vi "NML GPIB Data Log.vi"(0 "Point #":i32) -> (1 "GPIB Data":dbl[](array[numeric]) format="%.4e", 2 "Stop":bool)   [LabVIEW 2019]
doc: "VI which calls the appropriate GPIB routines for a variety of instruments.\nScott Hannahs, NHMFL-FSU, Nov. 1993"
uses:
  Sub Controls/Instrument.ctl
  Sub Controls/NML GPIB List.ctl
panel:
  in  "GPIB settings":T3={"#1"={"Instrument"=enum."None", "Instrument Address"="", "Parameters"=[]}, "#2"={"Instrument"=enum."None", "Instrument Address"="", "Parameters"=[]}, "#3"={"Instrument"=enum."None", "Instrument Address"="", "Parameters"=[]}, "#4"={"Instrument"=enum."None", "Instrument Address"="", "Parameters"=[]}, "#5"={"Instrument"=enum."None", "Instrument Address"="", "Parameters"=[]}, "#6"={"Instrument"=enum."None", "Instrument Address"="", "Parameters"=[]}, "#7"={"Instrument"=enum."None", "Instrument Address"="", "Parameters"=[]}, "#8"={"Instrument"=enum."None", "Instrument Address"="", "Parameters"=[]}, "#9"={"Instrument"=enum."None", "Instrument Address"="", "Parameters"=[]}, "#10"={"Instrument"=enum."None", "Instrument Address"="", "Parameters"=[]}, "#11"={"Instrument"=enum."None", "Instrument Address"="", "Parameters"=[]}, "#12"={"Instrument"=enum."None", "Instrument Address"="", "Parameters"=[]}, "#13"={"Instrument"=enum."None", "Instrument Address"="", "Parameters"=[]}, "#14"={"Instrument"=enum."None", "Instrument Address"="", "Parameters"=[]}, "#15"={"Instrument"=enum."None", "Instrument Address"="", "Parameters"=[]}, "#16"={"Instrument"=enum."None", "Instrument Address"="", "Parameters"=[]}, "#17"={"Instrument"=enum."None", "Instrument Address"="", "Parameters"=[]}, "#18"={"Instrument"=enum."None", "Instrument Address"="", "Parameters"=[]}, "#19"={"Instrument"=enum."None", "Instrument Address"="", "Parameters"=[]}, "#20"={"Instrument"=enum."Time Stamp", "Instrument Address"="", "Parameters"=[]}} {"#16"."Parameters" format="%.3e"; "#20"."Parameters" format="%.3e"; "#18"."Parameters" format="%.3e"; "#17"."Parameters" format="%.3e"; "#19"."Parameters" format="%.3e"; "#11"."Parameters" format="%.3e"; "#15"."Parameters" format="%.3e"; "#13"."Parameters" format="%.3e"; "#12"."Parameters" format="%.3e"; "#14"."Parameters" format="%.3e"; "#6"."Parameters" format="%.3e"; "#10"."Parameters" format="%.3e"; "#8"."Parameters" format="%.3e"; "#7"."Parameters" format="%.3e"; "#9"."Parameters" format="%.3e"; "#1"."Parameters" format="%.3e"; "#5"."Parameters" format="%.3e"; "#3"."Parameters" format="%.3e"; "#2"."Parameters" format="%.3e"; "#4"."Parameters" format="%.3e"}
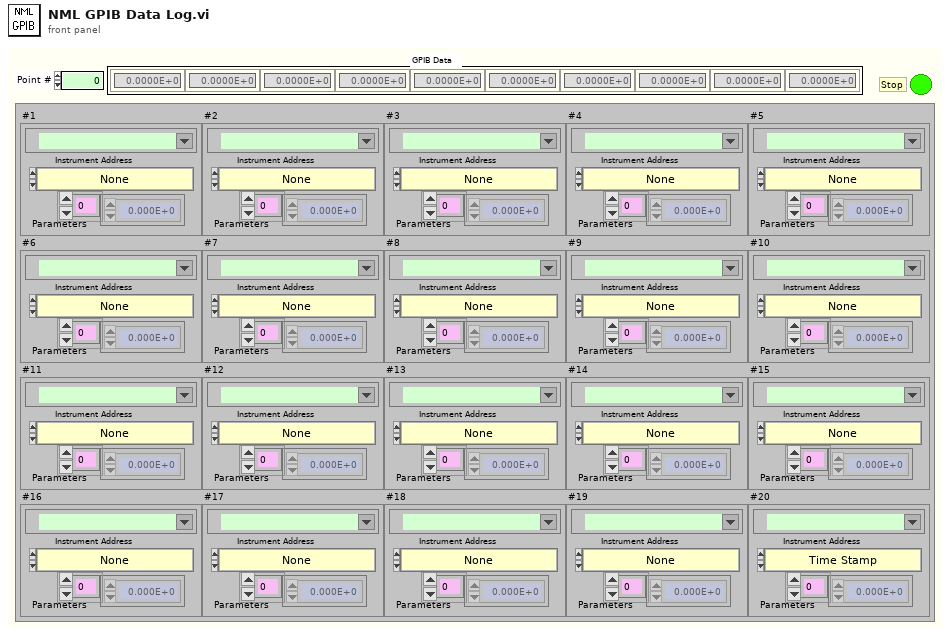
[diagram p1: front panel]
types:
  T1 = typedef "Instrument.ctl" = cluster{"Instrument":T2, "Instrument Address":refnum<visa-resource-name>, "Parameters":dbl[]}
  T2 = typedef "NML GPIB List.ctl" = enum16{"None", "Field", "Field - SCM1", "DMM", "DMM - HP 34401", "Keithley 2XXX", "Running DMM Ave", "Running HP34401", "Running K2XXX Ave", "SRS 830 - CH 1", "SRS 830 - CH1 & 2", "SRS PTC10", "Signal Rec 7265 - X", "Signal Rec 7265 - X&Y", "DRC 93C - Sample", "DRC 93C - Control", "DRC 93C - Sam&Con", "CryoCon Sensor A", "CryoCon Sensor B", "Cond 20C Sensor 1", "Cond 20C Sensor 2", "LS 336 Read", "LS 340 Read", "LS 370 Read", "LS 370 Select", "AVS 46 Bridge", "BLM Rotator Read Position", "Linear Research 700", "LR 700 Select", "Keithley 3330 - LCZ", "A-H Capacitance", "Digital Integrator", "SRS 400 Phot Ctr", "LakeShore VSM", "AMI He Level Meter", "Time Stamp", "Wait", "Invert Current", "K230 Linear V", "K230 VÅB^2", "Temp Ramp", "Power Ramp", "Freq Sweep", "LTC Stable T", "Scanner Step", "IMS Stepper Increment", "BLM Stepper Increment", "Omega CNi32"}
  T3 = cluster{"#1":T1, "#2":T1, "#3":T1, "#4":T1, "#5":T1, "#6":T1, "#7":T1, "#8":T1, "#9":T1, "#10":T1, "#11":T1, "#12":T1, "#13":T1, "#14":T1, "#15":T1, "#16":T1, "#17":T1, "#18":T1, "#19":T1, "#20":T1}
  T4 = cluster{"[0]":T1, "[1]":T1, "[2]":T1, "[3]":T1, "[4]":T1, "[5]":T1, "[6]":T1, "[7]":T1, "[8]":T1, "[9]":T1, "[10]":T1, "[11]":T1, "[12]":T1, "[13]":T1, "[14]":T1, "[15]":T1, "[16]":T1, "[17]":T1, "[18]":T1, "[19]":T1}
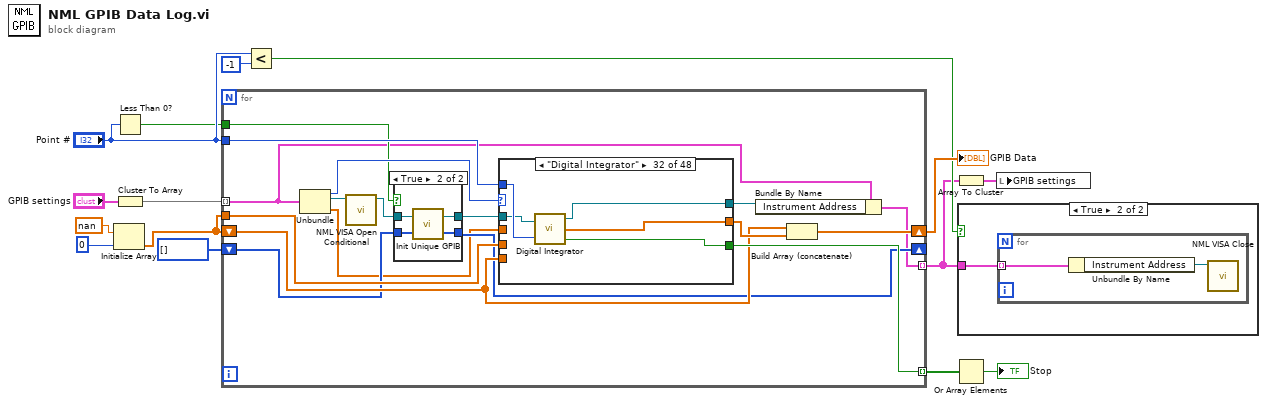
[diagram p0: block diagram]
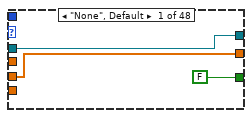
[diagram p4: hidden frame]
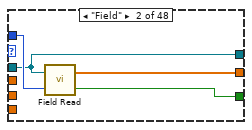
[diagram p5: hidden frame]
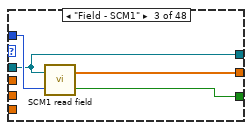
[diagram p6: hidden frame]
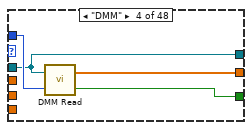
[diagram p7: hidden frame]
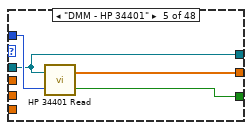
[diagram p8: hidden frame]
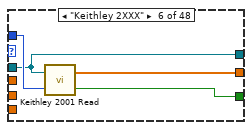
[diagram p9: hidden frame]
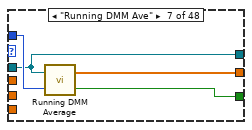
[diagram p10: hidden frame]
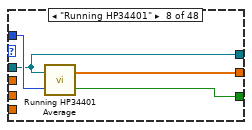
[diagram p11: hidden frame]
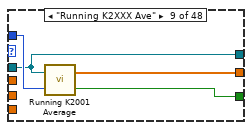
[diagram p12: hidden frame]
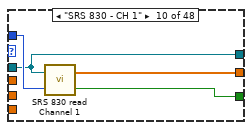
[diagram p13: hidden frame]
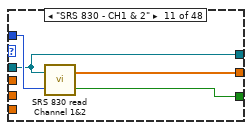
[diagram p14: hidden frame]
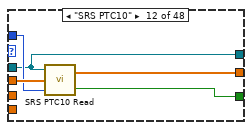
[diagram p15: hidden frame]
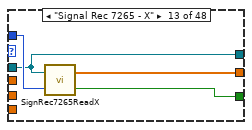
[diagram p16: hidden frame]
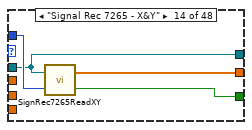
[diagram p17: hidden frame]
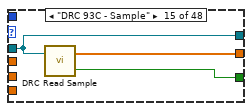
[diagram p18: hidden frame]
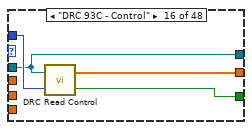
[diagram p19: hidden frame]
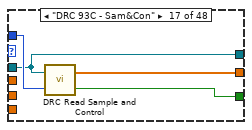
[diagram p20: hidden frame]
diagram:
  n1 = Initialize Array(nan, 0) -> (w5:dbl[])
  n2 = Less Than 0?(x="Point #") -> (x < 0?=w4:bool)
  n3 = Cluster To Array(cluster="GPIB settings") -> (array=w12:T1[])
  n4 = for {
    shift-right: [w32] -> w15
    shift-left: w5 -> [w27]
    tunnel: "Point #" -> [w23]
    tunnel: w12 -> [w21] mode=indexing
    tunnel: [w29] -> w11 mode=indexing
    tunnel: w5 -> [w28]
    tunnel: w4 -> [w22]
    shift-right: [w25] -> _
    shift-left: u16[] [] ("Inited dup") -> [w26]
    tunnel: [w20] -> w1 mode=indexing
    n5 = Unbundle(w21) -> ("Instrument"=w30:T2, "Instrument Address"=w16:refnum<visa-resource-name>, "Parameters"=w24:dbl[])
    n6 = call "NML VISA Open Conditional.vi"("VISA resource name"=w16) -> ("dup VISA Session"=w17:refnum<visa-resource-name>)  [unwired: 8 in, 2 out]
    n7 = case shown="True" w22 {
      tunnel: w26 -> [w33 w38]
      tunnel: [w33 w37] -> w25
      tunnel: w17 -> [w34 w36]
      tunnel: [w34 w35] -> w19
      frame False {
      }
      frame True {
        n8 = call "Init Unique GPIB.vi"("Inited"=w38, "VISA resource name"=w36) -> ("Inited dup"=w37:u16[], "dup VISA resource"=w35:refnum<visa-resource-name>)
      }
    }
    n9 = case shown="\"Digital Integrator\"" w30 {
      tunnel: [FALSE w44 w48 w52 w56 w60 w64 w68 w72 w77 w81 w83 w89 w93 w97 w101 w105 w108 w112 w116 w120 w124 w130 w135 w140 FALSE ("Stop") w149 w152 w156 w159 w163 w166 w172 w175 w179 w182 w187 w192 w197 w202 w207 w212 w217 w219 w225 w231 w233 w239] -> w29
      tunnel: w23 -> [_ w43 w47 w51 w55 w59 w63 w67 w71 w75 w79 w85 w88 w92 _ w99 w103 w107 w111 w115 w119 w125 w129 w133 w138 _ _ _ _ _ w161 w169 _ _ w177 w184 w189 w190 w194 w200 w205 w210 w215 w221 w226 w230 w235 _]
      tunnel: [w40 w45 w49 w53 w57 w61 w65 w69 w73 w76 w80 w84 w90 w94 w96 w100 w104 w109 w113 w117 w121 w123 w131 w136 w141 w145 w148 w151 w155 w158 w162 w167 w173 w176 w180 w183 w188 w193 w198 w203 w208 w213 w218 w220 w224 w232 w234 w240] -> w31
      tunnel: w19 -> [w39 w42 w46 w50 w54 w58 w62 w66 w70 w74 w78 w82 w87 w91 w95 w98 w102 w106 w110 w114 w118 w122 w127 w134 w139 w146 w150 w153 w157 w160 w164 w168 w171 w174 w178 w181 w185 w191 w196 w201 w206 w211 w216 w222 w227 w229 w237 w238]
      tunnel: w28 -> [w40 _ _ _ _ _ _ _ _ _ _ _ _ _ _ _ _ _ _ _ _ _ _ _ _ _ _ _ _ _ _ _ _ _ _ _ _ _ _ _ _ _ _ _ _ _ _ _]
      tunnel: w24 -> [_ _ _ _ _ _ _ _ _ _ _ w86 _ _ _ _ _ _ _ _ _ w126 w128 w132 w137 _ _ _ w154 _ _ _ w170 _ _ _ w186 _ w195 _ w204 w209 w214 _ w223 w228 w236 _]
      tunnel: w27 -> [_ _ _ _ _ _ _ _ _ _ _ _ _ _ _ _ _ _ _ _ _ _ _ _ _ _ _ _ _ _ _ _ _ _ _ _ _ _ _ w199 _ _ _ _ _ _ _ _]
      tunnel: [w39 w42 w46 w50 w54 w58 w62 w66 w70 w74 w78 w82 w87 w91 w95 w98 w102 w106 w110 w114 w118 w122 w127 w134 w139 w146 w150 w153 w157 w160 w164 w165 w171 w174 w178 w181 w185 w191 w196 w201 w206 w211 w216 w222 w227 w229 w237 w238] -> w18
      frame "None", Default {
      }
      frame "Field" {
        n10 = call "Field Read.vi"("Point #"=w43, "Instrument Address"=w42) -> ("Stop"=w44:bool, "Field"=w45:dbl[])
      }
      frame "Field - SCM1" {
        n11 = call "SCM1 read field.vi"("Point #"=w47, "Instrument Address"=w46) -> ("Stop"=w48:bool, "Output"=w49:dbl[])
      }
      frame "DMM" {
        n12 = call "DMM Read.vi"("Point #"=w51, "Instrument Address"=w50) -> ("Stop"=w52:bool, "Measurement"=w53:dbl[])
      }
      frame "DMM - HP 34401" {
        n13 = call "HP 34401 Read.vi"("Point #"=w55, "Instrument Address"=w54) -> ("Stop"=w56:bool, "Measurement"=w57:dbl[])
      }
      frame "Keithley 2XXX" {
        n14 = call "Keithley 2001 Read.vi"("Point #"=w59, "Instrument Address"=w58) -> ("Stop"=w60:bool, "Measurement"=w61:dbl[])
      }
      frame "Running DMM Ave" {
        n15 = call "Running DMM Average.vi"("Point #"=w63, "Instrument Address"=w62) -> ("Stop"=w64:bool, 1:w65:dbl[])
      }
      frame "Running HP34401" {
        n16 = call "Running HP34401 Average.vi"("Point #"=w67, "Instrument Address"=w66) -> ("Stop"=w68:bool, 1:w69:dbl[])
      }
      frame "Running K2XXX Ave" {
        n17 = call "Running K2001 Average.vi"("Point #"=w71, "Instrument Address"=w70) -> ("Stop"=w72:bool, 1:w73:dbl[])
      }
      frame "SRS 830 - CH 1" {
        n18 = call "SRS 830 read Channel 1.vi"("Point #"=w75, "Instrument Address"=w74) -> ("Stop"=w77:bool, "SRS 830 Output"=w76:dbl[])
      }
      frame "SRS 830 - CH1 & 2" {
        n19 = call "SRS 830 read Channel 1&2.vi"("Point #"=w79, "Instrument Address"=w78) -> ("Stop"=w81:bool, "SRS 830 Output"=w80:dbl[])
      }
      frame "SRS PTC10" {
        n20 = call "SRS PTC10 Read.vi"("Point #"=w85, "Parameters"=w86, "Instrument Address"=w82) -> ("Stop"=w83:bool, "Measurement"=w84:dbl[])
      }
      frame "Signal Rec 7265 - X" {
        n21 = call "SignRec7265ReadX.vi"("Point #"=w88, "Instrument Address"=w87) -> ("Stop"=w89:bool, "Measurement"=w90:dbl[])
      }
      frame "Signal Rec 7265 - X&Y" {
        n22 = call "SignRec7265ReadXY.vi"("Point #"=w92, "Instrument Address"=w91) -> ("Stop"=w93:bool, "Measurement"=w94:dbl[])
      }
      frame "DRC 93C - Sample" {
        n23 = call "DRC Read Sample.vi"("Instrument Address"=w95) -> ("Stop"=w97:bool, "Output"=w96:dbl[])  [unwired: 1 in]
      }
      frame "DRC 93C - Control" {
        n24 = call "DRC Read Control.vi"("Point #"=w99, "Instrument Address"=w98) -> ("Stop"=w101:bool, "Output"=w100:dbl[])
      }
      frame "DRC 93C - Sam&Con" {
        n25 = call "DRC Read Sample and Control.vi"("Point #"=w103, "Instrument Address"=w102) -> ("Stop"=w105:bool, "Output"=w104:dbl[])
      }
      frame "CryoCon Sensor A" {
        n26 = call "Cryocon read sensor 1.vi"("Point #"=w107, "Instrument Address"=w106) -> ("Stop"=w108:bool, "Output"=w109:dbl[])
      }
      frame "CryoCon Sensor B" {
        n27 = call "CryoCon read sensor 2.vi"("Point #"=w111, "Instrument Address"=w110) -> ("Stop"=w112:bool, "Output"=w113:dbl[])
      }
      frame "Cond 20C Sensor 1" {
        n28 = call "Conductus 20C read sensor 1.vi"("Point #"=w115, "Instrument Address"=w114) -> ("Stop"=w116:bool, "Output"=w117:dbl[])
      }
      frame "Cond 20C Sensor 2" {
        n29 = call "Conductus 20C read sensor 2.vi"("Point #"=w119, "Instrument Address"=w118) -> ("Stop"=w120:bool, "Output"=w121:dbl[])
      }
      frame "LS 336 Read" {
        n30 = call "LakeShore 336 Read.vi"("Point #"=w125, "Parameters"=w126, "Instrument Address"=w122) -> ("Stop"=w124:bool, "Measurement"=w123:dbl[])  [unwired: 1 in, 2 out]
      }
      frame "LS 340 Read" {
        n31 = call "LakeShore 340 Read.vi"("Point #"=w129, "Parameters"=w128, "Instrument Address"=w127) -> ("Stop"=w130:bool, "Measurement"=w131:dbl[])
      }
      frame "LS 370 Read" {
        n32 = call "LakeShore 370 Read.vi"("Point #"=w133, "Parameters"=w132, "Instrument Address"=w134) -> ("Stop"=w135:bool, "Measurement"=w136:dbl[])
      }
      frame "LS 370 Select" {
        n33 = call "LakeShore 370 Select Sensor.vi"("Point #"=w138, "Parameters"=w137, "Instrument Address"=w139) -> ("Stop"=w140:bool, "Array"=w141:dbl[])
      }
      frame "BLM Rotator Read Position" {
        n34 = call "BLM Read Position.vi"("Steps/rot"=8000.0, "Motor Address"="0", "Port Address"=w146) -> ("Response"=w147:dbl)  [unwired: 1 in, 3 out]
        n35 = Build Array(w147) -> (w145:dbl[])
      }
      frame "AVS 46 Bridge" {
        n36 = call "AVS46.vi"("Instrument Address"=w150) -> ("Stop"=w149:bool, "Measurement"=w148:dbl[])  [unwired: 1 in]
      }
      frame "Linear Research 700" {
        n37 = call "LR700 Read R.vi"("Instrument Address"=w153) -> ("Stop"=w152:bool, "Measurement"=w151:dbl[])  [unwired: 1 in]
      }
      frame "LR 700 Select" {
        n38 = call "LR700 Select Sensor.vi"("Parameters"=w154, "Instrument Address"=w157) -> ("Stop"=w156:bool, "Array"=w155:dbl[])
      }
      frame "Keithley 3330 - LCZ" {
        n39 = call "Keithley 3330 Read.vi"("Instrument Address"=w160) -> ("Stop"=w159:bool, "Measurement"=w158:dbl[])  [unwired: 1 in]
      }
      frame "A-H Capacitance" {
        n40 = call "A-H Cap.vi"("Point #"=w161, "Instrument Address"=w164) -> ("Stop"=w163:bool, "Measurement"=w162:dbl[])
      }
      frame "Digital Integrator" {
        n41 = call "Digital Integrator.vi"("Instrument Address"=w168, "Index"=w169) -> ("dup VISA Session"=w165:refnum<visa-resource-name>, 3:w167:dbl[], "Stop"=w166:bool)
      }
      frame "SRS 400 Phot Ctr" {
        n42 = call "SRS 400 Read.vi"("Parameters"=w170, "Instrument Address"=w171) -> ("Stop"=w172:bool, "Data"=w173:dbl[])
      }
      frame "LakeShore VSM" {
        n43 = call "LakeShore VSM 7300 EMU read.vi"("Instrument Address"=w174) -> ("Stop"=w175:bool, "Output"=w176:dbl[])  [unwired: 1 in]
      }
      frame "AMI He Level Meter" {
        n44 = call "AMI He Level.vi"("Point #"=w177, "Instrument Address"=w178) -> ("Stop"=w179:bool, "Measurement"=w180:dbl[])
      }
      frame "Time Stamp" {
        n45 = call "Time Stamp-old.vi"("Point #"=w184) -> ("Stop"=w182:bool, "Time Stamp (Sec)"=w183:dbl[])  [unwired: 1 in]
      }
      frame "Wait" {
        n46 = call "Seconds Wait.vi"("Point #"=w189, "Parameters"=w186) -> ("Stop"=w187:bool, "Time Stamp (Sec)"=w188:dbl[])
      }
      frame "Invert Current" {
        n47 = call "Invert Current Keithley 220.vi"("Point #"=w190, "Instrument Address"=w191) -> ("Stop"=w192:bool, "Keithley 220 Current"=w193:dbl[])  [unwired: 2 in]
      }
      frame "K230 Linear V" {
        n48 = call "Keithley 230 Voltage Ramp.vi"("Point #"=w194, "Parameters"=w195, "Instrument Address"=w196) -> ("Stop"=w197:bool, "Keithley 230 Voltage"=w198:dbl[])  [unwired: 1 in]
      }
      frame "K230 VÅB^2" {
        n49 = call "Keithley 230 V prop B^2.vi"("Point #"=w200, "GPIB Data In"=w199, "Instrument Address"=w201) -> ("Stop"=w202:bool, "Keithley 230 Voltage"=w203:dbl[])  [unwired: 1 in]
      }
      frame "Temp Ramp" {
        n50 = call "Conductus Ramp Temperature.vi"("Point #"=w205, "Parameters"=w204, "Instrument Address"=w206) -> ("Stop"=w207:bool, "Data Out"=w208:dbl[])  [unwired: 1 in]
      }
      frame "Power Ramp" {
        n51 = call "Conductus Ramp Power.vi"("Point #"=w210, "Parameters"=w209, "Instrument Address"=w211) -> ("Stop"=w212:bool, "Data Out"=w213:dbl[])  [unwired: 1 in]
      }
      frame "Freq Sweep" {
        n52 = call "SRS 830 Ramp Freq.vi"("Point #"=w215, "Parameters"=w214, "Instrument Address"=w216) -> ("Stop"=w217:bool, "Data Out"=w218:dbl[])  [unwired: 1 in]
      }
      frame "LTC Stable T" {
        n53 = call "LTC change to stable temp.vi"("Point Number"=w221, "L:TC 21 Address"=w222) -> ("Stop"=w219:bool, "Stable temperature (K)"=w220:dbl[])
      }
      frame "Scanner Step" {
        n54 = call "Scanme.vi"("Index"=w226, "Parameters"=w223, "Instrument Address"=w227) -> ("Stop"=w225:bool, "Array"=w224:dbl[])  [unwired: 1 in]
      }
      frame "IMS Stepper Increment" {
        n55 = call "IMS Stepper Control.vi"("Point #"=w230, "Parameters"=w228, "Instrument Address"=w229) -> ("Stop"=w231:bool, "Data Out"=w232:dbl[])  [unwired: 1 in]
      }
      frame "BLM Stepper Increment" {
        n56 = call "BLM control.vi"("Point #"=w235, "Parameters"=w236, "Instrument Address"=w237) -> ("Stop"=w233:bool, "Data Out"=w234:dbl[])  [unwired: 1 in]
      }
      frame "Omega CNi32" {
        n57 = call "Omega read sensor.vi"() -> ("Stop"=w239:bool, "Current Reading"=w240:dbl[])
      }
    }
    n58 = Bundle By Name(cluster=w21, "Instrument Address"=w18) -> (w20:T1)
    n59 = Build Array (concatenate)(w27, w31) -> (w32:dbl[])
  }
  "GPIB Data" <- w15
  n60 = Less?(x="Point #", y=-1) -> (x < y?=w2:bool)
  n61 = Array To Cluster(array=w1) -> (cluster=w10:T4)
  n62 = Or Array Elements(Boolean array=w11) -> (logical OR=→"Stop":bool)
  n63 = case shown="True" w2 {
    tunnel: w1 -> [_ w241]
    frame False {
    }
    frame True {
      n64 = for {
        tunnel: w241 -> [w243] mode=indexing
        n65 = Unbundle By Name(w243) -> ("Instrument Address"=w242:refnum<visa-resource-name>)
        n66 = call "NML VISA Close.vi"("VISA resource name"=w242) -> ()  [unwired: 10 in, 1 out]
      }
    }
  }
  n67 = local write "GPIB settings"(w10) -> ()
